vi "transfer_and_submit_job.vi"(7 "Date Folder":string, 8 "Password":string, 9 "Username":string, 10 "Remote Data Directory":string, 11 "Local Data Directory":string) -> ()   [LabVIEW 2014]
panel:
  out "standard error":string
  out "standard output":string
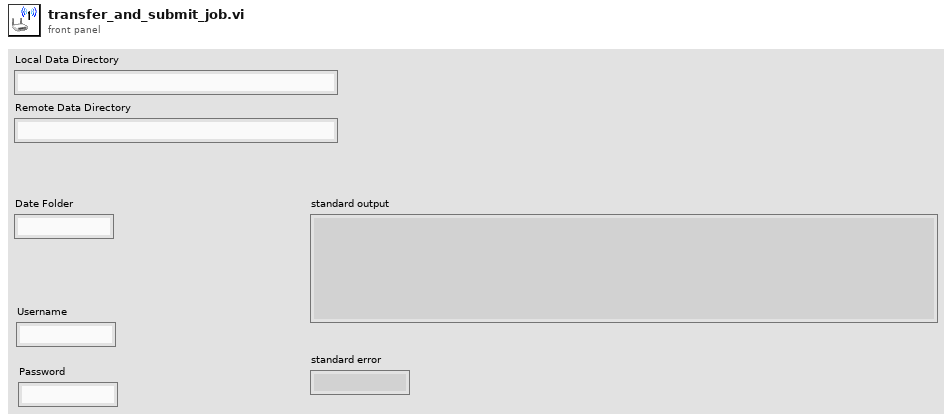
[diagram p1: front panel]
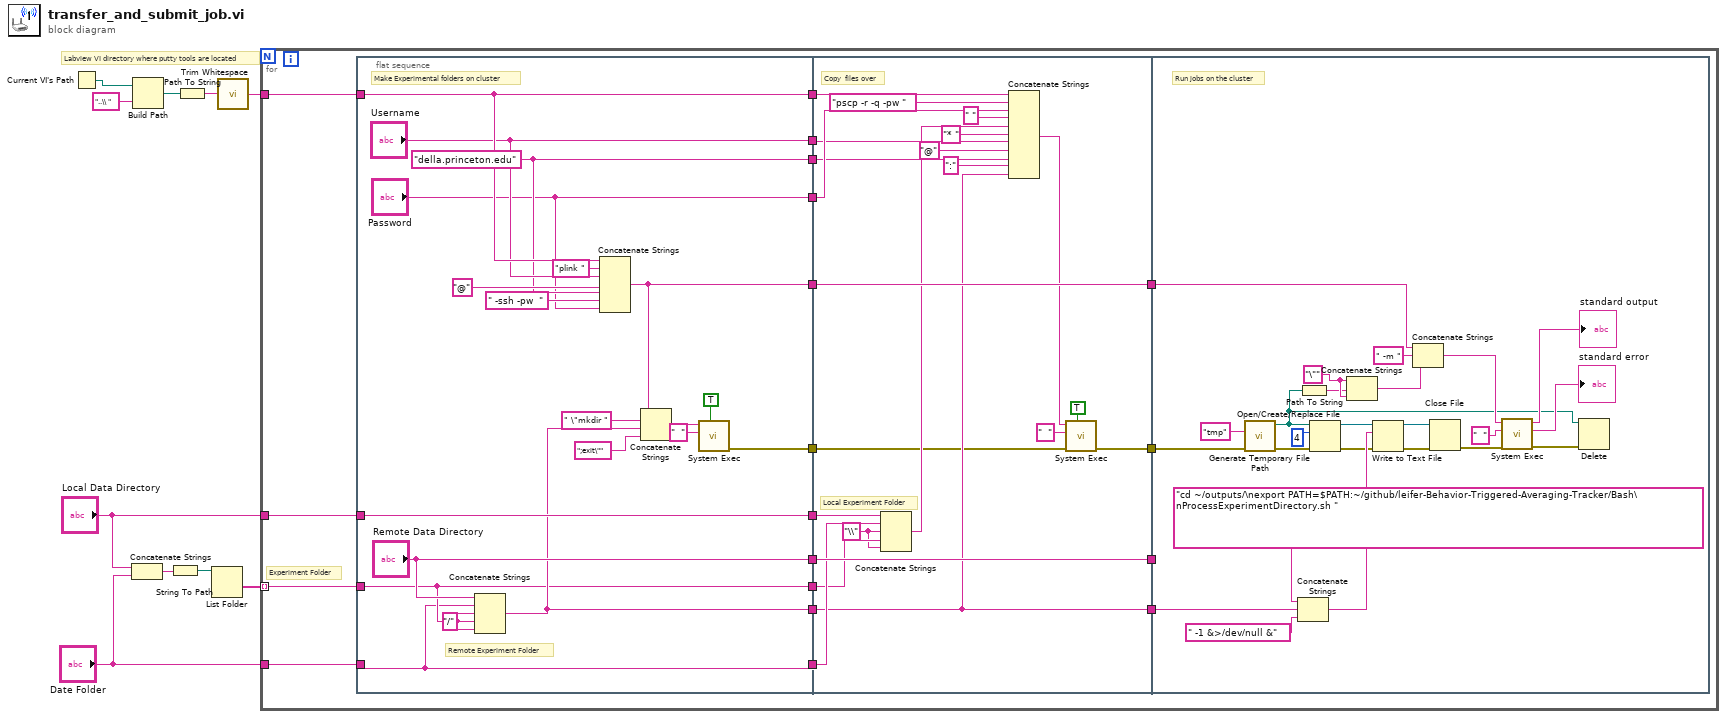
[diagram p0: block diagram]
diagram:
  # "Labview VI directory where putty tools are located"
  n1 = Current VI's Path() -> (path=w2:path)
  n2 = Concatenate Strings("Local Data Directory", "Date Folder") -> (w8:string)
  n3 = Build Path(base path=w2, name or relative path="..\\ ") -> (appended path=w4:path)
  n4 = String To Path(string=w8) -> (path=w7:path)
  n5 = Path To String(path=w4) -> (string=w5:string)
  n6 = List Folder(path=w7) -> (folder names=w6:string[])  [unwired: 3 in, 3 out]
  n7 = call <vilib>:"Trim Whitespace.vi"("string"=w5) -> ("trimmed string"=w1:string)  [unwired: 1 in]
  n8 = for {
    tunnel: "Date Folder" -> [w29]
    tunnel: "Local Data Directory" -> [w28]
    tunnel: w6 -> [w27] mode=indexing
    tunnel: w1 -> [w18]
    # "Experiment Folder"
    n9 = flat-sequence {
      tunnel: [w31] -> w25
      tunnel: w29 -> [w31]
      tunnel: w27 -> [w32]
      tunnel: [w32] -> w26
      tunnel: w28 -> [w41]
      tunnel: ["Remote Data Directory"] -> w24
      tunnel: ["Username"] -> w22
      tunnel: ["Password"] -> w21
      tunnel: [w43] -> w20
      tunnel: [w45] -> w19
      tunnel: w18 -> [w45]
      tunnel: [w41] -> w17
      tunnel: [w37] -> w15
      tunnel: [w34] -> w13
      tunnel: [w33] -> w12
      tunnel: w26 -> [w63]
      tunnel: w25 -> [w69]
      tunnel: w24 -> [w71]
      tunnel: [w71] -> w23
      tunnel: w22 -> [w58]
      tunnel: w21 -> [w65]
      tunnel: w20 -> [w57]
      tunnel: w19 -> [w66]
      tunnel: w17 -> [w70]
      tunnel: [w55] -> w16
      tunnel: w15 -> [w55]
      tunnel: [w68] -> w14
      tunnel: w13 -> [w68]
      tunnel: w12 -> [w51]
      tunnel: [w50] -> w11
      tunnel: w23 -> [_]
      tunnel: w16 -> [w74]
      tunnel: w14 -> [w73]
      tunnel: w11 -> [w72]
      frame #0 {
        w30 = "/"
        w43 = "della.princeton.edu"
        # "Remote Experiment Folder"
        # "Make Experimental folders on cluster"
        n10 = Concatenate Strings("Remote Data Directory", w31, w30, w32, w30) -> (w37:string)
        n11 = Concatenate Strings(w45, "plink ", "Username", "@", w43, " -ssh -pw  ", "Password") -> (w34:string)
        n12 = Concatenate Strings(w34, " \"mkdir ", w37, ";exit\"") -> (w35:string)
        n13 = call <vilib>:"System Exec.vi"("wait until completion? (T)"=TRUE, "standard input"="  ", "command line"=w35) -> ("error out"=w33:errorcluster)  [unwired: 5 in, 3 out]
      }
      frame #1 {
        w62 = "\\"
        # "Local Experiment Folder"
        # "Copy  files over"
        n14 = Concatenate Strings(w70, w69, w62, w63, w62) -> (w61:string)
        n15 = Concatenate Strings(w66, "pscp -r -q -pw ", w65, " ", w61, "* ", w58, "@", w57, ":", w55) -> (w52:string)
        n16 = call <vilib>:"System Exec.vi"("wait until completion? (T)"=TRUE, "error in (no error)"=w51, "standard input"="  ", "command line"=w52) -> ("error out"=w50:errorcluster)  [unwired: 4 in, 3 out]
      }
      frame #2 {
        w90 = "\""
        # "Run jobs on the cluster"
        n17 = call <vilib>:"Generate Temporary File Path.vi"("error in (no error)"=w72, "Temporary File Extension (tmp)"="tmp") -> ("error out"=w80:errorcluster, "Unique Temporary File Path"=w86:path)  [unwired: 8 in]
        n18 = Concatenate Strings("cd ~/outputs/\nexport PATH=$PATH:~/github/leifer-Behavior-Triggered-Averaging-Tracker/Bash\nProcessExperimentDirectory.sh ", w74, " -1 &>/dev/null &") -> (w88:string)
        n19 = Path To String(path=w86) -> (string=w89:string)
        n20 = Open/Create/Replace File(file path (use dialog)=w86, error in=w80, operation (0:open)=4) -> (refnum out=w81:refnum<file>, error out=w78:errorcluster)  [unwired: 3 in, 1 out]
        n21 = Concatenate Strings(w90, w89, w90) -> (w77:string)
        n22 = Write to Text File(file (use dialog)=w81, text=w88, error in=w78) -> (refnum out=w82:refnum<file>, error out=w79:errorcluster)  [unwired: 1 in, 1 out]
        n23 = Concatenate Strings(w73, " -m ", w77) -> (w91:string)
        n24 = Close File(refnum=w82, error in=w79) -> (error out=w83:errorcluster)  [unwired: 1 out]
        n25 = call <vilib>:"System Exec.vi"("error in (no error)"=w83, "standard input"="  ", "command line"=w91) -> ("error out"=w84:errorcluster, "standard error"=→"standard error":string, "standard output"=→"standard output":string)  [unwired: 5 in, 1 out]
        n26 = Delete(path (use dialog)=w86, error in=w84) -> ()  [unwired: 3 in, 3 out]
      }
    }
  }
